vi "SVA_MAIN_3.vi"() -> ()   [LabVIEW 2021]
uses:
  <vilib>/vision/NI_Vision_Development_Module.lvlib
panel:
  out "Cluster":T1
  in  "Control Points":u32=10
  out "BinT 2":T2(plugin-control) caption="Perfil lateral"
  out "BinP":T2(plugin-control) caption="Perfil lateral"
  in  "CrearPatrón":bool
  out "Pass Status":bool
  in  "Detener \nPrograma":bool
  in  "Max Distance 2":dbl=4.0 min=0.0 format="%.2f"
  out "Distance 2":dbl[](graph) caption="Distancia entre perfil ideal y perfil real"
  out "Perfil lateral":T2(plugin-control)
  in  "Lateral":bool
  in  "Max Distance":dbl=4.0 min=0.0 format="%.2f"
  out "Distance":dbl[](graph) caption="Distancia entre perfil ideal y perfil real"
  out "Perfil superior":T2(plugin-control)
  in  "Superior":bool
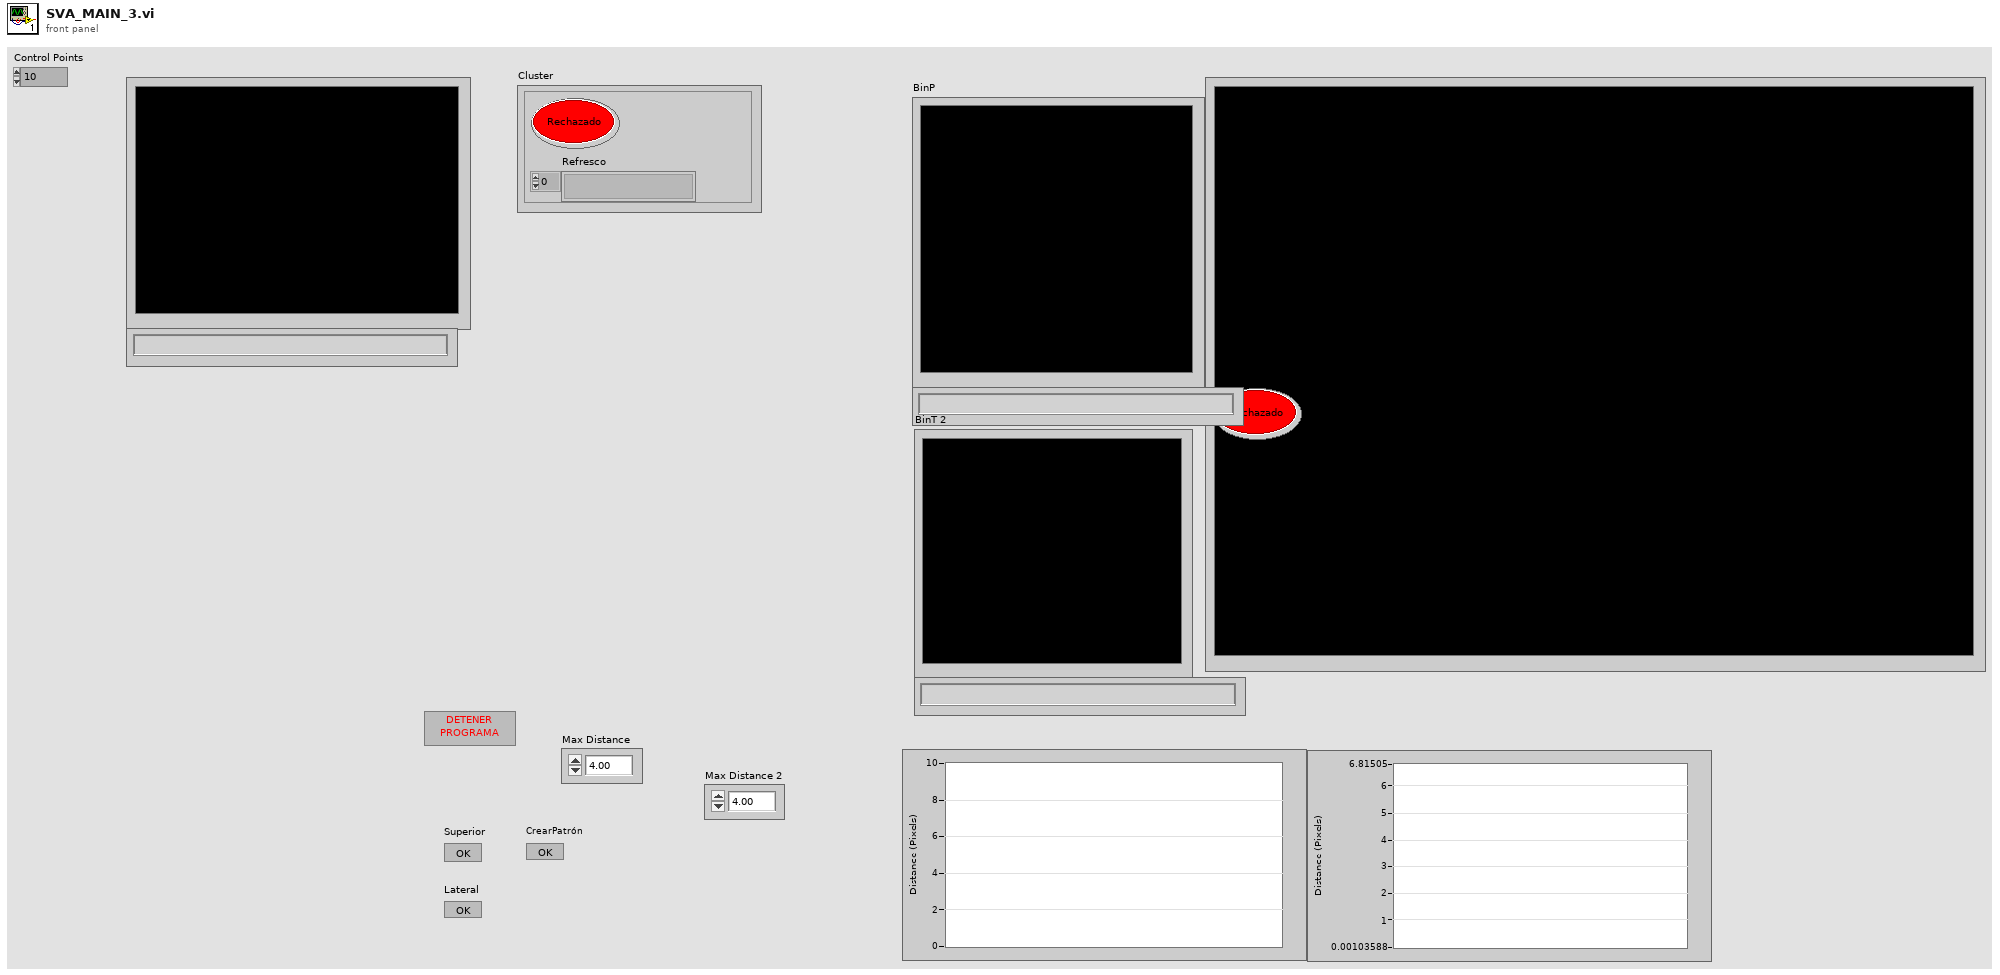
[diagram p1: front panel]
types:
  T1 = cluster{"Pass Status 2":bool, "Refresco":string[]}
  T2 = typedef "IMAQ Image.ctl" = refnum<image>
  T3 = enum16{"Rect Left To Right", "Rect Right To Left", "Rect Top To Bottom", "Rect Bottom To Top", "Annulus Inner To Outer", "Annulus Outer To Inner", "Annulus Start Angle To End Angle", "Annulus End Angle To Start Angle"}
  T4 = enum16{"Closest To Search Start", "Maximum Length", "Strongest Mean Gradient Change"}
  T5 = cluster{"Overlay?":bool, "Color":u32, "Width":u32, "Maintain Width?":bool}
  T6 = typedef "IMAQ Rectangle" = cluster{"Left":i32, "Top":i32, "Right":i32, "Bottom":i32, "Rotation":dbl}
  T7 = typedef "ROI Descriptor" = cluster{"Global Rectangle":i32[], "Contours":cluster{"ID":enum32{"External", "Internal"}, "Type":u32, "Coordinates":i32[]}[]}
  T8 = cluster{"Target Point":cluster{"X":dbl, "Y":dbl}, "Template Point":cluster{"X":dbl, "Y":dbl}, "Distance":dbl}[]
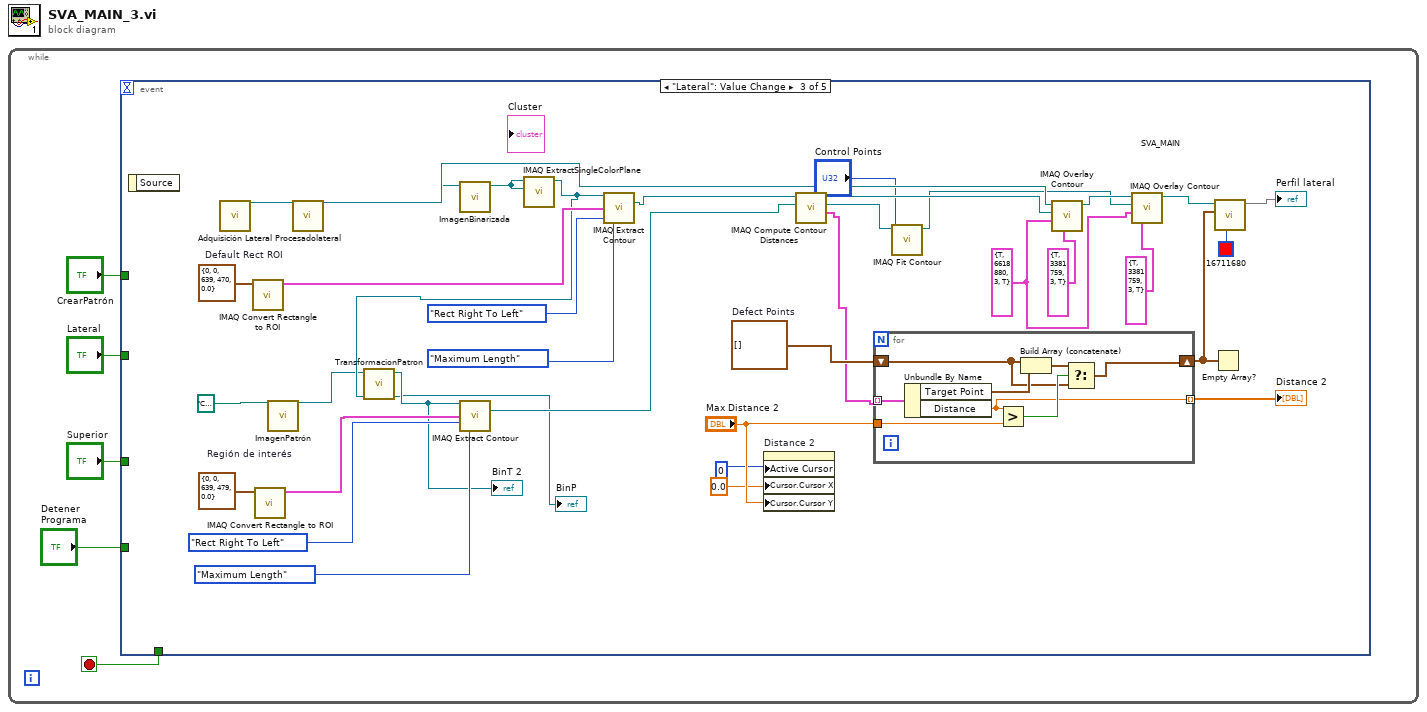
[diagram p0: block diagram]
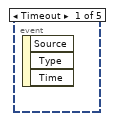
[diagram p2: hidden frame]
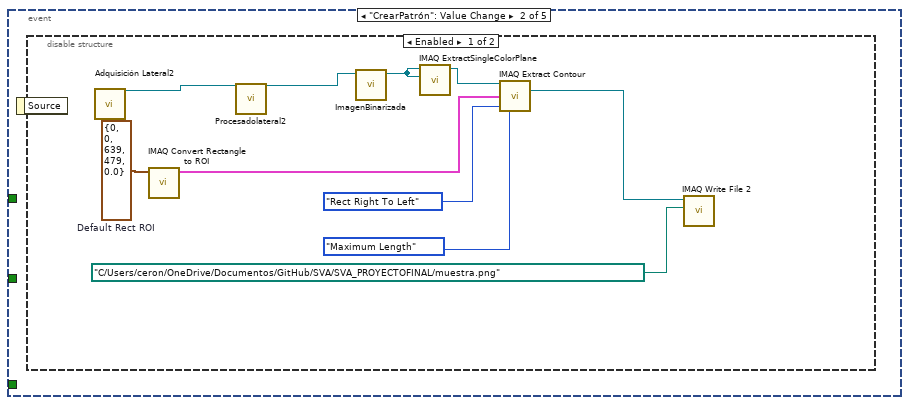
[diagram p3: hidden frame]
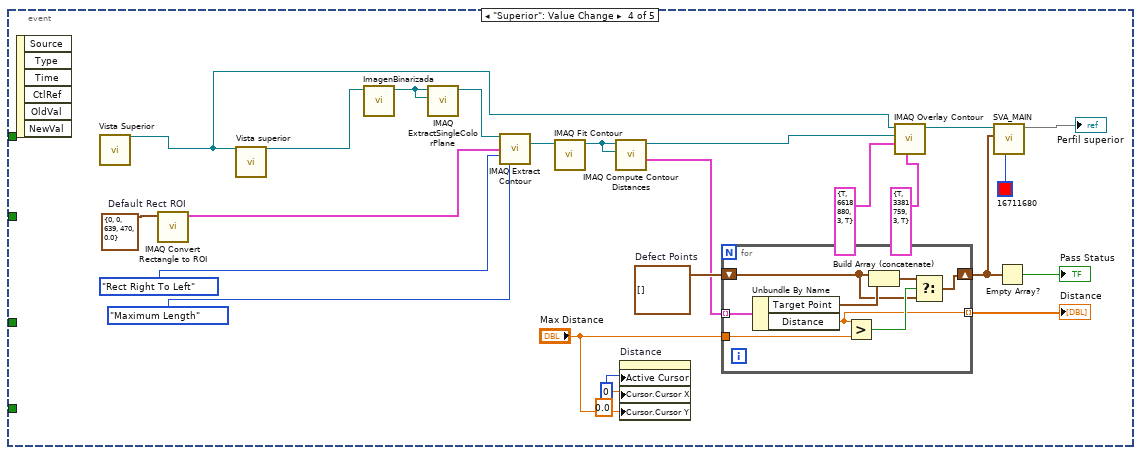
[diagram p5: hidden frame]
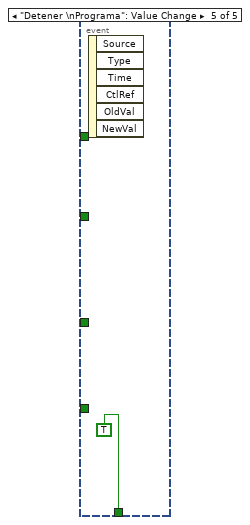
[diagram p6: hidden frame]
diagram:
  n1 = while {
    stop <- w1 stop-if-true
    n2 = event shown="[2] \"Lateral\": Value Change" {
      selector: _ -> [_ _ _ _ _]
      dyn-events: _ -> [_ _ _ _ _]
      timeout: _ -> [_ _ _ _ _]
      tunnel: "Superior" -> [_ _ _ _ _]
      tunnel: "Lateral" -> [_ _ _ _ _]
      tunnel: "CrearPatrón" -> [_ _ _ _ _]
      tunnel: "Detener \nPrograma" -> [_ _ _ _ _]
      tunnel: [_ _ _ _ TRUE] -> w1
      event Timeout {
        n3 = event-data() -> ()  [unwired: 1 in, 3 out]
      }
      event "CrearPatrón": Value Change {
        n4 = event-data() -> ()  [unwired: 1 in, 1 out]
        n5 = disable-structure shown="Enabled" {
          frame Enabled {
            w11 = T6 {"Left"=0, "Top"=0, "Right"=639, "Bottom"=479, "Rotation"=0.0}  # Default Rect ROI
            n6 = call "Adquisición Lateral2"() -> ("Image Out"=w7:T2)  [unwired: 26 in, 1 out]
            n7 = call "IMAQ Convert Rectangle to ROI"("Rectangle"=w11) -> ("ROI Descriptor"=w10:T7)  [unwired: 8 in, 1 out]
            n8 = call "Procesadolateral2"("Image In"=w7) -> ("Image Out"=w6:T2)  [unwired: 25 in, 1 out]
            n9 = call "ImagenBinarizada.vi"("Refnum in"=w6) -> ("Refnum out"=w14:T2)  [unwired: 10 in]
            n10 = call "IMAQ ExtractSingleColorPlane"("Image Dst"=w14, "Image Src"=w14) -> ("Image Dst Out"=w15:T2)  [unwired: 8 in, 1 out]
            n11 = call "IMAQ Extract Contour"("Source Image"=w15, "ROI Descriptor"=w10, "Search Direction"=T3."Rect Right To Left", "Contour Selection"=T4."Maximum Length") -> ("Contour Image Out"=w9:T2)  [unwired: 4 in, 7 out]
            n12 = call-poly "IMAQ Write File 2"("File Path"=path "C:/Users/ceron/OneDrive/Documentos/GitHub/SVA/SVA_PROYECTOFINAL/muestra.png" ("Imagen \nPatrón 2"), "Image"=w9) -> ()  [unwired: 8 in, 2 out]
          }
          frame Disabled {
          }
        }
      }
      event "Lateral": Value Change {
        w37 = T6 {"Left"=0, "Top"=0, "Right"=639, "Bottom"=479, "Rotation"=0.0}  # Región de interés
        w40 = T6 {"Left"=0, "Top"=0, "Right"=639, "Bottom"=470, "Rotation"=0.0}  # Default Rect ROI
        w47 = cluster{"X":dbl, "Y":dbl}[] []  # Defect Points
        w22 = T5 {"Overlay?"=TRUE, "Color"=6618880, "Width"=3, "Maintain Width?"=TRUE} ("Contour Points Settings")
        n13 = event-data() -> ()  [unwired: 1 in, 1 out]
        n14 = call "Adquisición Lateral"() -> ("Image Out"=w53:T2)  [unwired: 26 in, 1 out]
        n15 = call "IMAQ Convert Rectangle to ROI"("Rectangle"=w40) -> ("ROI Descriptor"=w39:T7)  [unwired: 8 in, 1 out]
        n16 = call "IMAQ Convert Rectangle to ROI"("Rectangle"=w37) -> ("ROI Descriptor"=w34:T7)  [unwired: 8 in, 1 out]
        n17 = call "ImagenPatrón"("Image Path"=path "C:/Users/ceron/OneDrive/Documentos/GitHub/SVA/SVA_PROYECTOFINAL/muestra.png" ("Imagen \nPatrón")) -> ("Image Out"=w17:T2)  [unwired: 25 in, 1 out]
        n18 = call "Procesadolateral"("Image In"=w53) -> ("Image Out"=w41:T2, "Classes (TipoRefresco)"=w33:string[])  [unwired: 23 in, 2 out]
        n19 = call "ImagenBinarizada.vi"("Refnum in"=w41) -> ("Refnum out"=w21:T2)  [unwired: 10 in]
        n20 = call "IMAQ ExtractSingleColorPlane"("Image Dst"=w21, "Image Src"=w21) -> ("Image Dst Out"=w18:T2)  [unwired: 8 in, 1 out]
        n21 = call "TransformacionPatron.vi"("Patrón original"=w18, "Toma original"=w17) -> ("Patron Original"=→"BinP":T2, "Toma corregida"=w20:T2)  [unwired: 8 in]
        "BinT 2" <- w20
        n22 = call "IMAQ Extract Contour"("Source Image"=w20, "ROI Descriptor"=w34, "Search Direction"=T3."Rect Right To Left", "Contour Selection"=T4."Maximum Length") -> ("Contour Image Out"=w31:T2)  [unwired: 4 in, 7 out]
        n23 = call "IMAQ Extract Contour"("Source Image"=w18, "ROI Descriptor"=w39, "Search Direction"=T3."Rect Right To Left", "Contour Selection"=T4."Maximum Length") -> ("Contour Image Out"=w32:T2)  [unwired: 4 in, 7 out]
        n24 = property on="Distance 2" class="WFGraph (strict)"("Active Cursor"=u32 0, "Cursor.Cursor X"=0.0 ("Cursor.Cursor Position:Cursor X"), "Cursor.Cursor Y"="Max Distance 2") -> ()  [unwired: 2 in, 2 out]
        n25 = call "IMAQ Compute Contour Distances"("Template Contour Image"=w31, "Target Contour Image"=w32) -> ("Distances"=w29:T8, "Template Contour Image Out (dup)"=w28:T2, "Target Contour Image Out (dup)"=w26:T2)  [unwired: 3 in, 4 out]
        n26 = for {
          tunnel: w29 -> [w54] mode=indexing
          shift-right: [w57] -> w50
          shift-left: w47 -> [w58]
          tunnel: [w56] -> w30 mode=indexing
          tunnel: "Max Distance 2" -> [w55]
          n27 = Unbundle By Name(w54) -> ("Target Point"=w61:cluster{"X":dbl, "Y":dbl}, "Distance"=w56:dbl)
          n28 = Greater?(x=w56, y=w55) -> (0:w60:bool)
          n29 = Build Array (concatenate)(w58, w61) -> (w59:cluster{"X":dbl, "Y":dbl}[])
          n30 = Select(t=w59, s=w60, f=w58) -> (s? t:f=w57:cluster{"X":dbl, "Y":dbl}[])
        }
        "Distance 2" <- w30
        n31 = call-poly "IMAQ Fit Contour"("Control Points"="Control Points", "Contour Image"=w28) -> ("Contour Image Out"=w25:T2)  [unwired: 2 in, 7 out]
        n32 = call "IMAQ Overlay Contour"("Contour Equation Settings"=T5 {"Overlay?"=TRUE, "Color"=3381759, "Width"=3, "Maintain Width?"=TRUE}, "Contour Points Settings"=w22, "Contour Image"=w26, "Image"=w53) -> ("Image Out"=w27:T2)  [unwired: 2 in, 5 out]
        n33 = call "IMAQ Overlay Contour"("Contour Equation Settings"=T5 {"Overlay?"=TRUE, "Color"=3381759, "Width"=3, "Maintain Width?"=TRUE}, "Contour Points Settings"=w22, "Contour Image"=w25, "Image"=w27) -> ("Image Out"=w24:T2)  [unwired: 2 in, 5 out]
        n34 = Empty Array?(array=w50) -> (empty?=w51:bool)
        n35 = call "SVA_MAIN.vi"(6:u32 16711680 ("Color"), 10:w50, 11:w24) -> (3:→"Perfil lateral")  [unwired: 8 in]
      }
      event "Superior": Value Change {
        w65 = T6 {"Left"=0, "Top"=0, "Right"=639, "Bottom"=470, "Rotation"=0.0}  # Default Rect ROI
        w76 = cluster{"X":dbl, "Y":dbl}[] []  # Defect Points
        n36 = event-data() -> ()  [unwired: 1 in, 6 out]
        n37 = call "Vista Superior"() -> ("Image Out"=w62:T2)  [unwired: 26 in, 1 out]
        n38 = call "IMAQ Convert Rectangle to ROI"("Rectangle"=w65) -> ("ROI Descriptor"=w64:T7)  [unwired: 8 in, 1 out]
        n39 = call "Vista superior"("Image In"=w62) -> ("Image Out"=w63:T2)  [unwired: 25 in, 1 out]
        n40 = call "ImagenBinarizada.vi"("Refnum in"=w63) -> ("Refnum out"=w68:T2)  [unwired: 10 in]
        n41 = call "IMAQ ExtractSingleColorPlane"("Image Dst"=w68, "Image Src"=w68) -> ("Image Dst Out"=w69:T2)  [unwired: 8 in, 1 out]
        n42 = call "IMAQ Extract Contour"("Source Image"=w69, "ROI Descriptor"=w64, "Search Direction"=T3."Rect Right To Left", "Contour Selection"=T4."Maximum Length") -> ("Contour Image Out"=w84:T2)  [unwired: 4 in, 7 out]
        n43 = call-poly "IMAQ Fit Contour"("Contour Image"=w84) -> ("Contour Image Out"=w74:T2)  [unwired: 3 in, 7 out]
        n44 = call "IMAQ Compute Contour Distances"("Template Contour Image"=w74, "Target Contour Image"=w74) -> ("Distances"=w75:T8, "Target Contour Image Out (dup)"=w85:T2)  [unwired: 3 in, 5 out]
        n45 = property on="Distance" class="WFGraph (strict)"("Active Cursor"=u32 0, "Cursor.Cursor X"=0.0 ("Cursor.Cursor Position:Cursor X"), "Cursor.Cursor Y"="Max Distance") -> ()  [unwired: 2 in, 2 out]
        n46 = for {
          tunnel: w75 -> [w93] mode=indexing
          shift-right: [w88] -> w81
          shift-left: w76 -> [w89]
          tunnel: [w87] -> w80 mode=indexing
          tunnel: "Max Distance" -> [w86]
          n47 = Unbundle By Name(w93) -> ("Target Point"=w92:cluster{"X":dbl, "Y":dbl}, "Distance"=w87:dbl)
          n48 = Greater?(x=w87, y=w86) -> (0:w91:bool)
          n49 = Build Array (concatenate)(w89, w92) -> (w90:cluster{"X":dbl, "Y":dbl}[])
          n50 = Select(t=w90, s=w91, f=w89) -> (s? t:f=w88:cluster{"X":dbl, "Y":dbl}[])
        }
        "Distance" <- w80
        n51 = call "IMAQ Overlay Contour"("Contour Equation Settings"=T5 {"Overlay?"=TRUE, "Color"=3381759, "Width"=3, "Maintain Width?"=TRUE}, "Contour Points Settings"=T5 {"Overlay?"=TRUE, "Color"=6618880, "Width"=3, "Maintain Width?"=TRUE}, "Contour Image"=w85, "Image"=w62) -> ("Image Out"=w77:T2)  [unwired: 2 in, 5 out]
        n52 = call "SVA_MAIN.vi"(6:u32 16711680 ("Color"), 10:w81, 11:w77) -> (3:→"Perfil superior")  [unwired: 8 in]
        n53 = Empty Array?(array=w81) -> (empty?=→"Pass Status":bool)
      }
      event "Detener \nPrograma": Value Change {
        n54 = event-data() -> ()  [unwired: 1 in, 6 out]
      }
    }
  }
